vi "01-31-17.vi"() -> ()   [LabVIEW 2016]
panel:
  out "XY Graph 8":cluster{dbl[], dbl[]}[](graph)
  out "XY Graph 7":cluster{dbl[], dbl[]}[](graph)
  out "XY Graph 6":cluster{dbl[], dbl[]}[](graph)
  out "XY Graph 5":cluster{dbl[], dbl[]}[](graph)
  out "XY Graph 4":cluster{dbl[], dbl[]}[](graph)
  out "XY Graph 3":cluster{dbl[], dbl[]}[](graph)
  out "XY Graph 2":cluster{dbl[], dbl[]}[](graph)
  out "XY Graph":cluster{dbl[], dbl[]}[](graph)
  # "Dual bane separated test"
  # "1x"
  # "2x"
  # "4x"
  # "Colson 3600"
  # "^^^ (@.9 pos DS)"
  # "^^^ (Back to 1)"
  # "^^^"
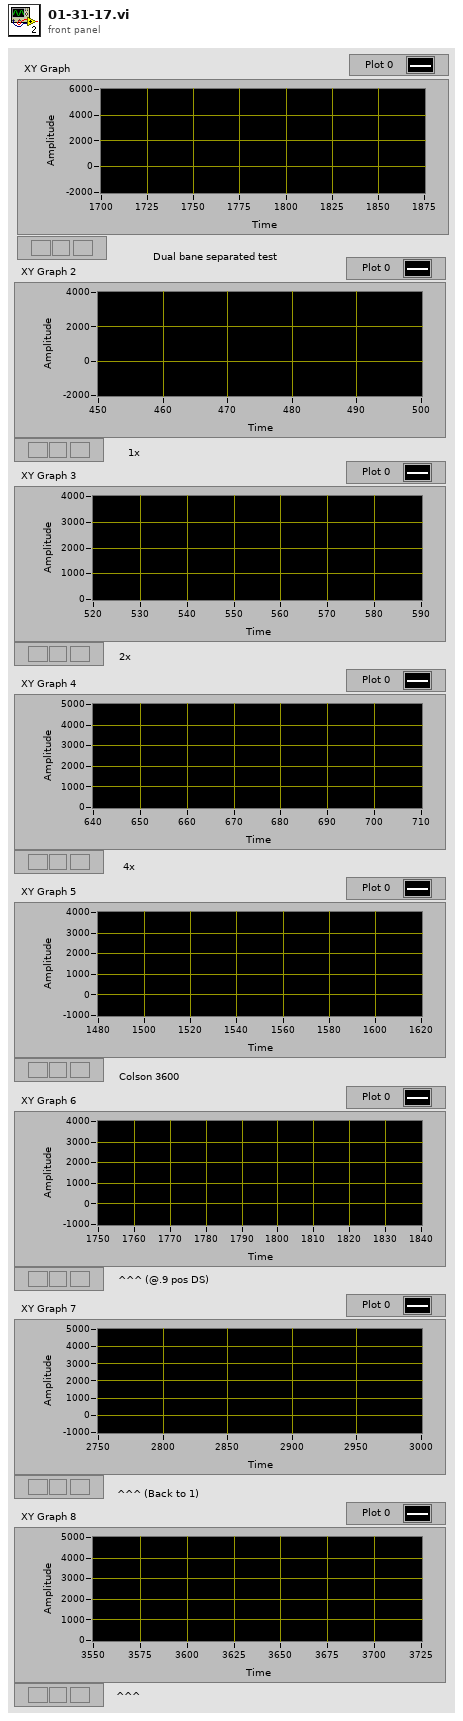
[diagram p1: front panel]
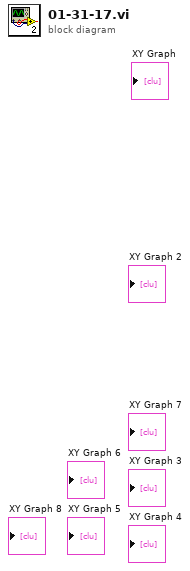
[diagram p0: block diagram]
diagram:
